vi "Get 1553 Message Data.vi"(0 "MSG DATA":u16[](array[numeric]), 5 "1553 Parameter":T1, 11 "error in (no error)":errorcluster) -> (4 "Value":dbl, 15 "error out":errorcluster)   [LabVIEW 2014, in "AIT 1553 Custom Device.lvlib"]
uses:
  AIT 1553 Custom Device.lvlib
  Controls/1553 Param.ctl
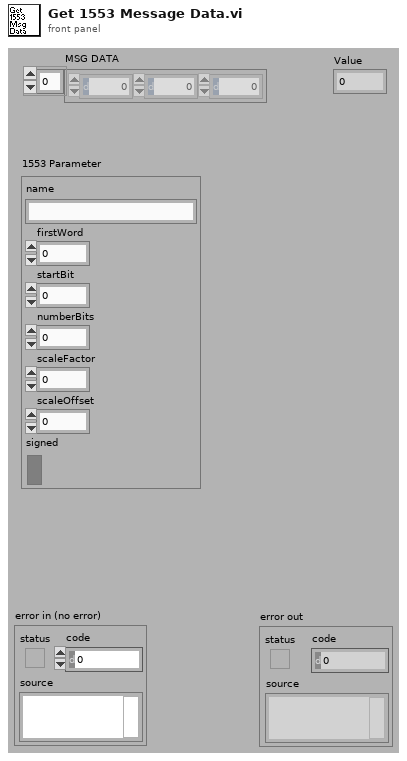
[diagram p1: front panel]
types:
  T1 = typedef "AIT 1553 Custom Device.lvlib/1553 Param.ctl" = cluster{"name":string, "firstWord":i32, "startBit":i32, "numberBits":i32, "scaleFactor":dbl, "scaleOffset":dbl, "signed":bool}
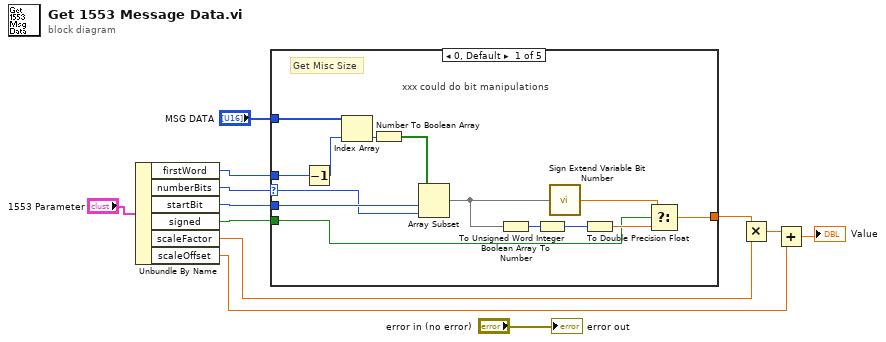
[diagram p0: block diagram]
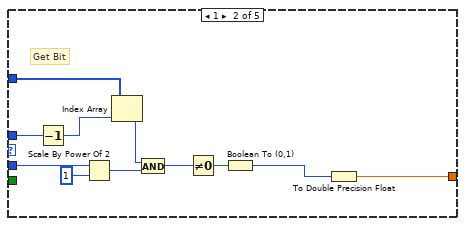
[diagram p2: hidden frame]
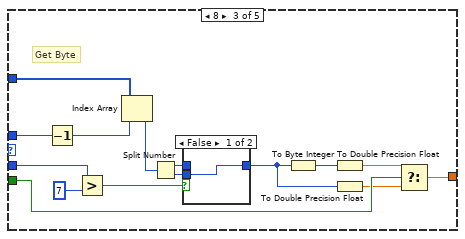
[diagram p3: hidden frame]
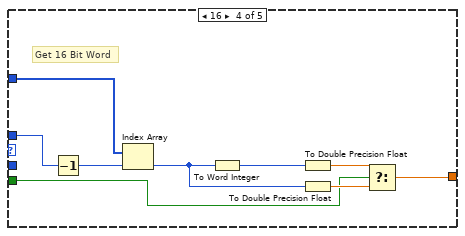
[diagram p5: hidden frame]
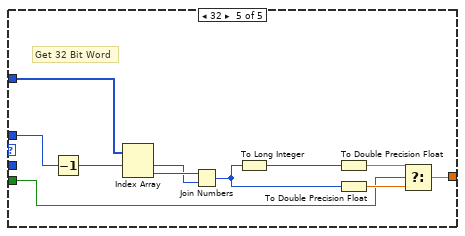
[diagram p6: hidden frame]
diagram:
  n1 = Unbundle By Name("1553 Parameter") -> ("firstWord"=w9:i32, "numberBits"=w8:i32, "startBit"=w7:i32, "signed"=w2:bool, "scaleFactor"=w5:dbl, "scaleOffset"=w4:dbl)
  n2 = case shown="0, Default" w8 {
    selector: w8 -> [w20 _ _ _ _]
    tunnel: "MSG DATA" -> [w24 w36 w52 w62 w72]
    tunnel: w9 -> [w26 w37 w51 w63 w74]
    tunnel: w7 -> [w21 w30 w45 _ _]
    tunnel: w2 -> [w17 _ w41 w55 w66]
    tunnel: [w16 w27 w38 w57 w67] -> w1
    frame 0, Default {
      # "xxx could do bit manipulations"
      # "Get Misc Size"
      n3 = Decrement(x=w26) -> (x-1=w23:i32)
      n4 = Index Array(array=w24, index=w23) -> (element=w25:u16)
      n5 = Number To Boolean Array(number=w25) -> (Boolean array=w22:bool[])
      n6 = Array Subset(array=w22, index=w21, length=w20) -> (w14:bool[])
      n7 = Boolean Array To Number(Boolean array=w14) -> (number=w15:u32)
      n8 = To Unsigned Word Integer(number=w15) -> (unsigned 16bit integer=w18:u16)
      n9 = call "Sign Extend Variable Bit Number.vi"("Variable Bit Number"=w14) -> ("Sign extended value"=w13:dbl)  [unwired: 14 in]
      n10 = To Double Precision Float(number=w18) -> (double precision float=w19:dbl)
      n11 = Select(t=w13, s=w17, f=w19) -> (s? t:f=w16:dbl)
    }
    frame 1 {
      # "Get Bit"
      n12 = Decrement(x=w37) -> (x-1=w33:i32)
      n13 = Scale By Power Of 2(n=w30, x=u16 1) -> (x*2^n=w35:u16)
      n14 = Index Array(array=w36, index=w33) -> (element=w34:u16)
      n15 = And(x=w34, y=w35) -> (x .and. y?=w29:u16)
      n16 = Not Equal To 0?(x=w29) -> (x != 0?=w31:bool)
      n17 = Boolean To (0,1)(Boolean=w31) -> (0, 1=w28:i16)
      n18 = To Double Precision Float(number=w28) -> (double precision float=w27:dbl)
    }
    frame 8 {
      # "Get Byte"
      n19 = Decrement(x=w51) -> (x-1=w44:i32)
      n20 = Greater?(x=w45, y=u16 7) -> (0:w48:bool)
      n21 = Index Array(array=w52, index=w44) -> (element=w49:u16)
      n22 = Split Number(x=w49) -> (hi(x)=w47:u8, lo(x)=w46:u8)
      n23 = case shown="False" w48 {
        tunnel: w47 -> [_ w54]
        tunnel: w46 -> [w53 _]
        tunnel: [w53 w54] -> w42
        frame False {
        }
        frame True {
        }
      }
      n24 = To Byte Integer(number=w42) -> (8bit integer=w43:i8)
      n25 = To Double Precision Float(number=w43) -> (double precision float=w40:dbl)
      n26 = To Double Precision Float(number=w42) -> (double precision float=w39:dbl)
      n27 = Select(t=w40, s=w41, f=w39) -> (s? t:f=w38:dbl)
    }
    frame 16 {
      # "Get 16 Bit Word"
      n28 = Decrement(x=w63) -> (x-1=w61:i32)
      n29 = Index Array(array=w62, index=w61) -> (element=w58:u16)
      n30 = To Word Integer(number=w58) -> (16bit integer=w56:i16)
      n31 = To Double Precision Float(number=w56) -> (double precision float=w60:dbl)
      n32 = To Double Precision Float(number=w58) -> (double precision float=w59:dbl)
      n33 = Select(t=w60, s=w55, f=w59) -> (s? t:f=w57:dbl)
    }
    frame 32 {
      # "Get 32 Bit Word"
      n34 = Decrement(x=w74) -> (x-1=w73:i32)
      n35 = Index Array(array=w72, index #1=w73) -> (element #1=w70:u16, element #2=w71:u16)  [unwired: 1 in]
      n36 = Join Numbers(hi=w71, lo=w70) -> ((hi.lo)=w64:u32)
      n37 = To Long Integer(number=w64) -> (32bit integer=w65:i32)
      n38 = To Double Precision Float(number=w65) -> (double precision float=w69:dbl)
      n39 = To Double Precision Float(number=w64) -> (double precision float=w68:dbl)
      n40 = Select(t=w69, s=w66, f=w68) -> (s? t:f=w67:dbl)
    }
  }
  n41 = Multiply(x=w1, y=w5) -> (x*y=w6:dbl)
  n42 = Add(x=w6, y=w4) -> (x+y=→"Value":dbl)
  "error out" <- "error in (no error)"
